vi "Get Data.vi"(0 "OphirFastX":refnum<k7>, 1 "Notifier":refnum<notifier>, 3 "Timeout (ms)":i32) -> (6 "Data":dbl[](array[numeric]), 9 "Error":errorcluster)   [LabVIEW 2009]
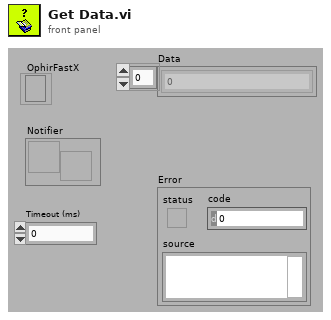
[diagram p1: front panel]
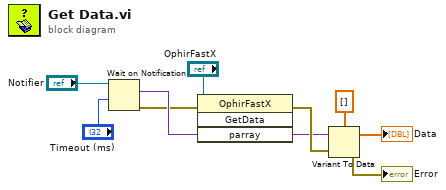
[diagram p0: block diagram]
diagram:
  n1 = Wait on Notification(notifier="Notifier", timeout in ms (-1)="Timeout (ms)") -> (notification=w7:variant, error out=w6:errorcluster)  [unwired: 2 in, 2 out]
  n2 = invoke class="OphirFastX" method="GetData"(reference="OphirFastX", error in=w6, "parray"=w7) -> (error out=w4:errorcluster, "parray"=w3:variant)  [unwired: 1 in, 2 out]
  n3 = Variant To Data(error in=w4, Variant=w3, type=dbl[] []) -> (error out=→"Error":errorcluster, data=→"Data":dbl[])
